vi "多值分割.vi"() -> (0 "确定":bool, 2 "个数":u8, 3 "阈值数组":T1(array[cluster]) {"Replace Value" format="%.2f"; "Upper value" format="%.2f"; "Lower value" format="%.2f"}, 5 "自动":bool)   [LabVIEW 2018]
panel:
  in  "分割数":u8
  in  "阈值数组":T1(array[cluster]) {"Replace Value" format="%.2f"; "Upper value" format="%.2f"; "Lower value" format="%.2f"}
  in  "自动":bool
  in  "确定":bool
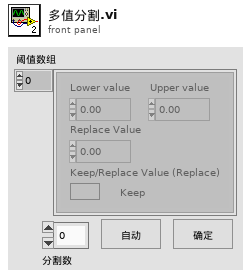
[diagram p1: front panel]
types:
  T1 = cluster{"Lower value":sgl, "Upper value":sgl, "Replace Value":sgl, "Keep/Replace Value (Replace)":bool}[]
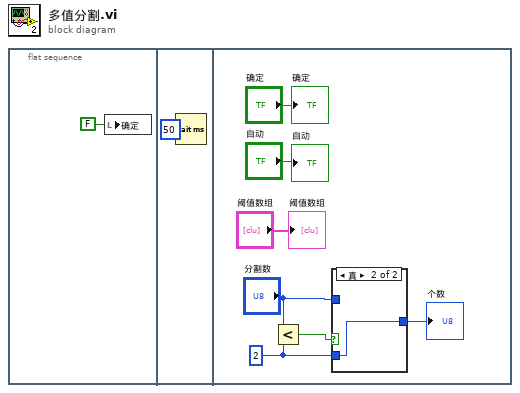
[diagram p0: block diagram]
diagram:
  n1 = flat-sequence {
    frame #0 {
      n2 = local write "确定"(FALSE ("确定")) -> ()
    }
    frame #1 {
      n3 = Wait (ms)(milliseconds to wait=u32 50 ("等待时间（毫秒）")) -> ()  [unwired: 1 out]
    }
    frame #2 {
      w4 = u8 2 ("y")
      n4 = Less?(x="分割数", y=w4) -> (x < y?=w6:bool)
      n5 = case shown="真" w6 {
        tunnel: "分割数" -> [w10 _]
        tunnel: w4 -> [_ w11]
        tunnel: [w10 w11] -> w3
        frame False {
        }
        frame True {
        }
      }
      "个数" <- w3
      "确定" <- "确定"
      "自动" <- "自动"
      "阈值数组" <- "阈值数组"
    }
  }
